vi "MessdatenAuslesen.vi"(6 "Faktor2 (1)":dbl=1.0, 7 "Points":i32=250, 8 "error in":errorcluster, 9 "Timeout (10000)":u32=10000, 10 "Source Channel (0: Channel 1)":i32(ring) items=["Channel 1"=0, "Channel 2"=1, "Channel 3"=2, "Channel 4"=3, "Waveform Memory 1"=5, "Waveform Memory 2"=6, "Serial Bus 1"=7, "Serial Bus 2"=8, "Digital Bus Low"=9, "Digital Bus High "=10, "Digital Bus 1"=11, "Digital Bus 2"=12, "Function 1"=32, "Function 2"=33, "Function 3"=34, "Function 4"=35, "Math 1"=36, "Math 2"=37, "Math 3"=38, "Math 4"=39], 11 "VISA Name OZ in(OZ)":refnum<visa-resource-name>="USB0::0x0957::0x179B::MY54313507::INSTR") -> (0 "error out":errorcluster, 1 "Messdaten":dbl[](array[numeric]), 2 "Waveform Data":waveform(dbl)(graph), 3 "VISA resource name out":refnum<visa-resource-name>)   [LabVIEW 2016]
doc: "Gibt die aufgenommenen Oszilloskop-Daten des gewählten Kanals zurück. Anschliesend wird bei den Messdaten noch der Offset des Oszilloskop abezogen.\nDie Aufnahme wird in einem vorherigen VI initialisiert."
panel:
  out "Anzahl ausgelesener Punkte":string
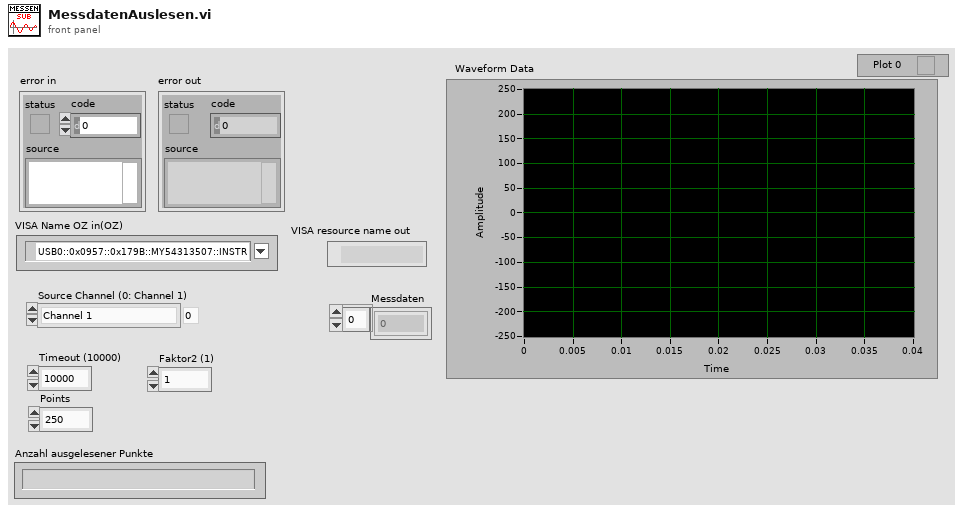
[diagram p1: front panel]
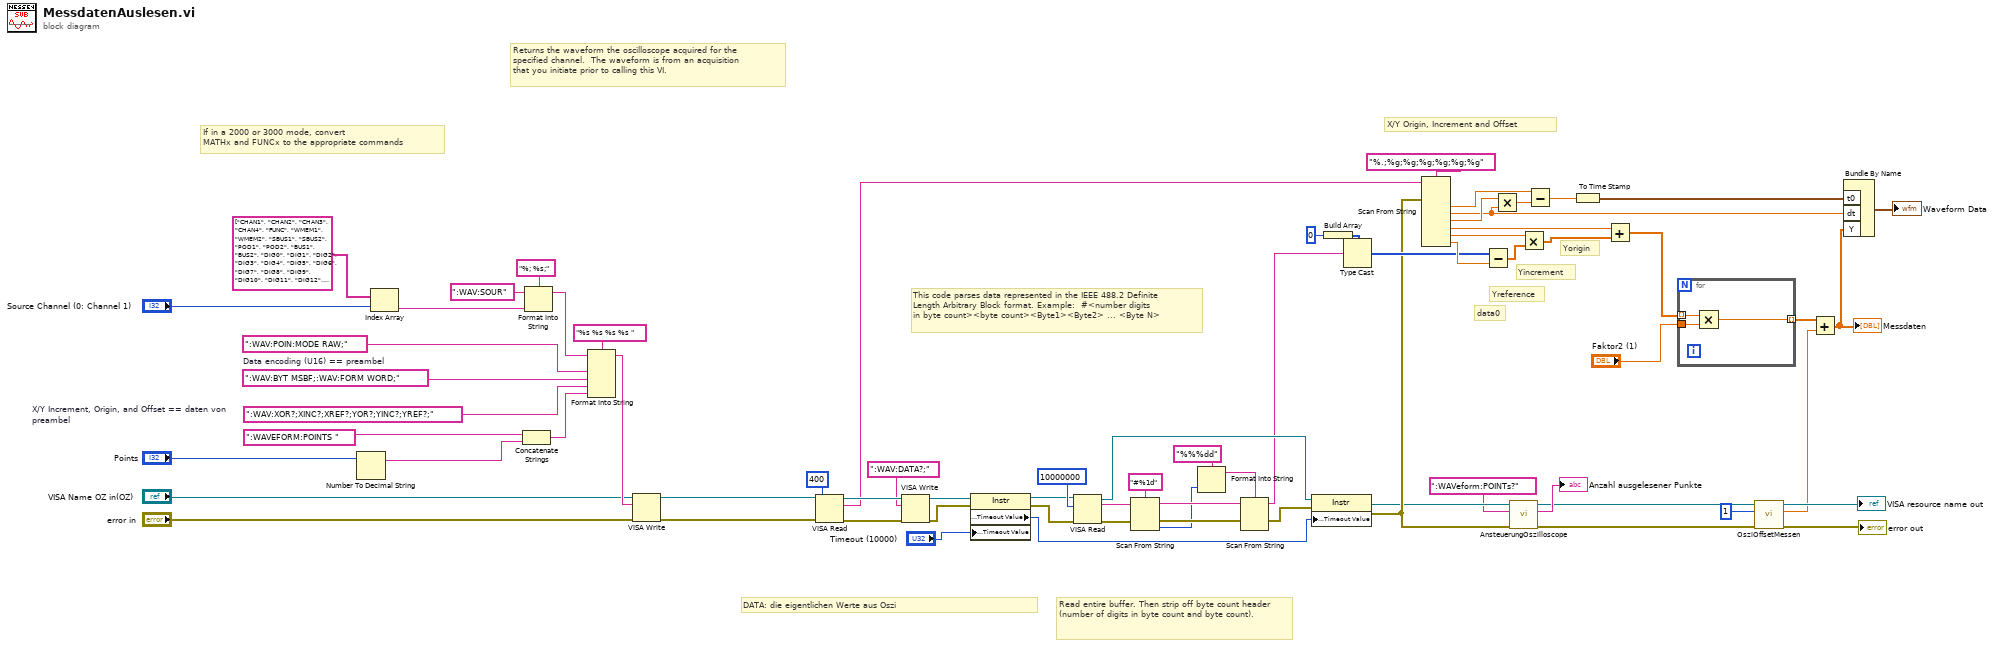
[diagram p0: block diagram]
diagram:
  w24 = ":WAV:XOR?;XINC?;XREF?;YOR?;YINC?;YREF?;"  # X/Y Increment, Origin, and Offset == daten von preambel
  w34 = ":WAV:BYT MSBF;:WAV:FORM WORD;"  # Data encoding (U16) == preambel
  # "Yorigin"
  # "data0"
  # "Yreference"
  # "Yincrement"
  # "DATA: die eigentlichen Werte aus Oszi"
  # "If in a 2000 or 3000 mode, convert\nMATHx and FUNCx to the appropriate commands"
  # "Read entire buffer. Then strip off byte count header (number of digits in byte count and byte count)."
  # "This code parses data represented in the IEEE 488.2 Definite \nLength Arbitrary Block format. Example:  #<number digits \nin byte count><byte count><Byte1><Byte2> ... <Byte N>"
  # "X/Y Origin, Increment and Offset"
  # "Returns the waveform the oscilloscope acquired for the \nspecified channel.  The waveform is from an acquisition \nthat you initiate prior to calling this VI."
  n1 = Number To Decimal String(number="Points") -> (decimal integer string=w17:string)  [unwired: 1 in]
  n2 = Index Array(array=string[] ["CHAN1", "CHAN2", "CHAN3", "CHAN4", "FUNC", "WMEM1", "WMEM2", "SBUS1", "SBUS2", "POD1", "POD2", "BUS1", "BUS2", "DIG0", "DIG1", "DIG2", "DIG3", "DIG4", "DIG5", "DIG6", "DIG7", "DIG8", "DIG9", "DIG10", "DIG11", "DIG12", "DIG13", "DIG14", "DIG15", "EXT", "LINE", "WGEN", "FUNC1", "FUNC2", "FUNC3", "FUNC4", "MATH1", "MATH2", "MATH3", "MATH4"], index="Source Channel (0: Channel 1)") -> (element=w31:string)
  n3 = Concatenate Strings(":WAVEFORM:POINTS " ("Eingang 4"), w17) -> (w18:string)
  n4 = Format Into String(format string="%; %s;", initial string=":WAV:SOUR" ("Eingangs-String"), w31) -> (resulting string=w22:string)  [unwired: 1 in, 1 out]
  n5 = Format Into String(format string="%s %s %s %s ", initial string=w22, ":WAV:POIN:MODE RAW;", w34, w24, w18) -> (resulting string=w21:string)  [unwired: 1 in, 1 out]
  n6 = VISA Write(VISA resource name="VISA Name OZ in(OZ)", write buffer=w21, error in (no error)="error in") -> (VISA resource name out=w38:refnum<visa-resource-name>, error out=w37:errorcluster)  [unwired: 1 out]
  n7 = VISA Read(VISA resource name=w38, byte count=u32 400, error in (no error)=w37) -> (VISA resource name out=w55:refnum<visa-resource-name>, read buffer=w16:string, error out=w54:errorcluster)  [unwired: 1 out]
  n8 = VISA Write(VISA resource name=w55, write buffer=":WAV:DATA?;", error in (no error)=w54) -> (VISA resource name out=w56:refnum<visa-resource-name>, error out=w57:errorcluster)  [unwired: 1 out]
  n9 = property class="Instr"(reference=w56, error in=w57, "General Settings:Timeout Value"="Timeout (10000)") -> (reference out=w51:refnum<visa-resource-name>, error out=w50:errorcluster, "General Settings:Timeout Value"=w53:u32)
  n10 = VISA Read(VISA resource name=w51, byte count=u32 10000000, error in (no error)=w50) -> (VISA resource name out=w49:refnum<visa-resource-name>, read buffer=w60:string, error out=w58:errorcluster)  [unwired: 1 out]
  n11 = Scan From String(format string="#%1d", input string=w60, error in=w58) -> (remaining string=w64:string, error out=w62:errorcluster, output 1=w61:i32)  [unwired: 1 in, 2 out]
  n12 = Format Into String(format string="%%%dd", w61) -> (resulting string=w63:string)  [unwired: 2 in, 1 out]
  n13 = Scan From String(format string=w63, input string=w64, error in=w62) -> (remaining string=w11:string, error out=w46:errorcluster)  [unwired: 1 in, 3 out]
  n14 = property class="Instr"(reference=w49, error in=w46, "General Settings:Timeout Value"=w53) -> (reference out=w29:refnum<visa-resource-name>, error out=w30:errorcluster)
  n15 = Build Array(u16 0) -> (w48:u16[])
  n16 = Type Cast(type=w48, x=w11) -> (*(type *) &x=w43:u16[])
  n17 = Scan From String(format string="%.;%g;%g;%g;%g;%g;%g", input string=w16, error in=w30) -> (output 1=w13:dbl, output 2=w14:dbl, output 3=w69:dbl, output 4=w40:dbl, output 5=w42:dbl, output 6=w44:dbl)  [unwired: 1 in, 9 out]
  n18 = Subtract(x=w43, y=w44) -> (x-y=w41:dbl[])
  n19 = Multiply(x=w69, y=w14) -> (x*y=w67:dbl)
  n20 = call "AnsteuerungOszilloscope.vi"("Error_in"=w30, "Eingangs-String"=":WAVeform:POINTs?" ("format string"), "VISA Name OZ in(OZ)"=w29) -> ("Error_out"=w7:errorcluster, "Ausgangs-String"=→"Anzahl ausgelesener Punkte":string, "VISA Name OZ out"=w9:refnum<visa-resource-name>)  [unwired: 6 in]
  n21 = Multiply(x=w42, y=w41) -> (x*y=w39:dbl[])
  n22 = Subtract(x=w13, y=w67) -> (x-y=w68:dbl)
  n23 = To Time Stamp(1:w68) -> (0:w70:timestamp)
  n24 = Add(x=w40, y=w39) -> (x+y=w3:dbl[])
  n25 = for {
    tunnel: w3 -> [w75] mode=indexing
    tunnel: "Faktor2 (1)" -> [w74]
    tunnel: [w73] -> w2 mode=indexing
    n26 = Multiply(x=w75, y=w74) -> (x*y=w73:dbl)
  }
  n27 = call "OsziOffsetMessen.vi"("Error_in"=w7, "Channel"=1, "VISA Name OZ in(OZ)"=w9) -> ("Error_out"=→"error out":errorcluster, "Offset_Spannung"=w4:dbl, "VISA Name OZ out"=→"VISA resource name out":refnum<visa-resource-name>)  [unwired: 6 in]
  n28 = Add(x=w2, y=w4) -> (x+y=w1:dbl[])
  "Messdaten" <- w1
  n29 = Bundle By Name("t0"=w70, "dt"=w14, "Y"=w1) -> (→"Waveform Data":waveform(dbl))  [unwired: 1 out]
